vi "Full_Adder.vi"() -> ()   [LabVIEW 2024]
panel:
  out "carry":bool
  out "sum":bool
  in  "C":bool
  in  "B":bool
  in  "A":bool
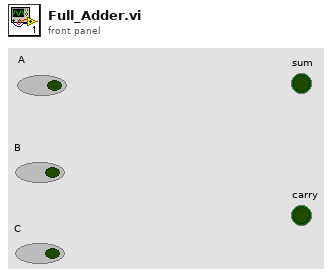
[diagram p1: front panel]
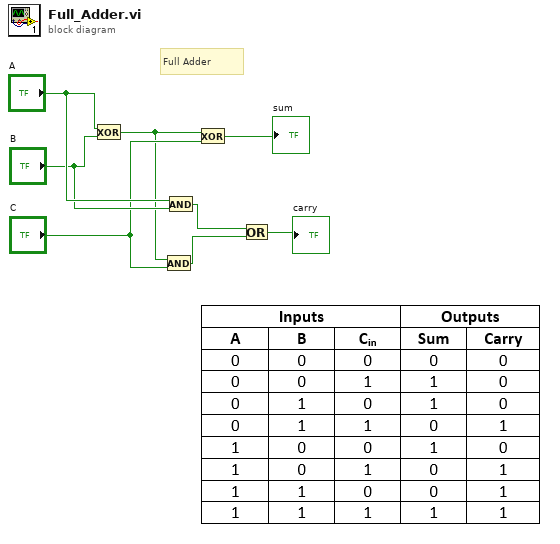
[diagram p0: block diagram]
diagram:
  # "Full Adder"
  n1 = Exclusive Or(1:"B", 2:"A") -> (0:w5:bool)
  n2 = And(x=w5, y="C") -> (x .and. y?=w3:bool)
  n3 = And(x="A", y="B") -> (x .and. y?=w4:bool)
  n4 = Exclusive Or(1:"C", 2:w5) -> (0:→"sum":bool)
  n5 = Or(x=w4, y=w3) -> (x .or. y?=→"carry":bool)
